vi "Test Wav Write.vi"() -> ()   [LabVIEW 2015]
uses:
  File IO VIs/Wave File VIs/Wave-EPL Chunk Variable.ctl
  <vilib>/sound2/lvsound2.llb/Sound Data Format.ctl
  <vilib>/sound2/lvsound2.llb/Sound File Write Open.vi
  <vilib>/sound2/lvsound2.llb/Sound File Write (DBL Single).vi
  <vilib>/Analysis/NI_AALBase.lvlib
panel:
  out "error out":errorcluster
  in  "EPL Variables":T1[](array[typedef])
  in  "path":path=path "C:/Experiment VIs/Utility VIs/Test VIs/test.wav"
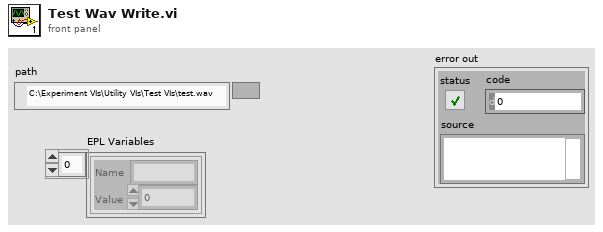
[diagram p1: front panel]
types:
  T1 = typedef "Wave-EPL Chunk Variable.ctl" = cluster{"Name":string, "Value":dbl}
  T2 = typedef "Sound Data Format.ctl" = cluster{"sample rate (S/s)":dbl, "number of channels":i32, "bits per sample":i32}
  T3 = enum16{"open", "replace", "create", "open or create", "replace or create", "replace or create with confirmation"}
  T4 = typedef "Sound File Refnum.ctl" = refnum<file>
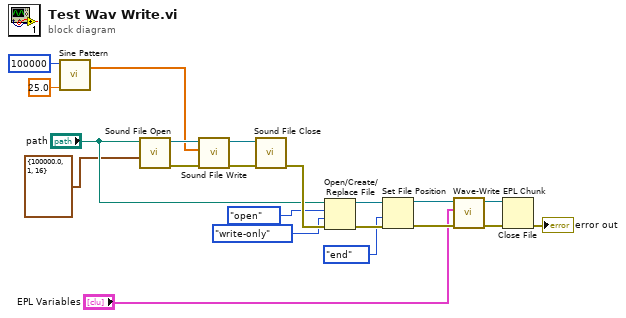
[diagram p0: block diagram]
diagram:
  n1 = call <vilib>:"Sine Pattern.vi"("cycles"=25.0, "samples"=100000) -> ("Sinusoidal Pattern"=w16:dbl[])  [unwired: 2 in, 1 out]
  n2 = call-poly <vilib>:"Sound File Open.vi"("sound format"=T2 {"sample rate (S/s)"=100000.0, "number of channels"=1, "bits per sample"=16}, "path"="path") -> ("error out"=w19:errorcluster, "sound file refnum"=w18:T4)  [unwired: 8 in]
  n3 = call-poly <vilib>:"Sound File Write.vi"("error in (no error)"=w19, "data"=w16, "sound file refnum"=w18) -> ("error out"=w17:errorcluster, "sound file refnum out"=w14:T4)  [unwired: 7 in]
  n4 = call <vilib>:"Sound File Close.vi"("error in (no error)"=w17, "sound file refnum"=w14) -> ("error out"=w15:errorcluster)  [unwired: 9 in]
  n5 = Open/Create/Replace File(file path (use dialog)="path", error in=w15, operation (0:open)=T3."open", access (0:read/write)=enum16{"read/write", "read-only", "write-only"}."write-only") -> (refnum out=w11:refnum<file>, error out=w12:errorcluster)  [unwired: 2 in, 1 out]
  n6 = Set File Position(refnum=w11, from (0:start)=enum16{"start", "end", "current"}."end", error in=w12) -> (refnum out=w7:refnum<file>, error out=w6:errorcluster)  [unwired: 1 in]
  n7 = call "Wave-Write EPL Chunk.vi"("error in (no error)"=w6, "EPL Variables"="EPL Variables", "refnum"=w7) -> ("error out"=w4:errorcluster, "refnum out"=w3:refnum<file>)  [unwired: 7 in]
  n8 = Close File(refnum=w3, error in=w4) -> (error out=→"error out":errorcluster)  [unwired: 1 out]
